vi "MaineReal.vi"() -> ()   [LabVIEW 2013]
panel:
  in  "AirmarVISAReference":refnum<visa-resource-name>="COM1"
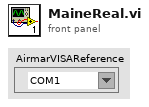
[diagram p1: front panel]
types:
  T1 = typedef "Notifiers.ctl" = cluster{"BoatSpeed":refnum<notifier>, "WindSpeed":refnum<notifier>, "MainPosition":refnum<notifier>, "JibPosition":refnum<notifier>, "MissionCheckOff":refnum<notifier>, "EStop":refnum<notifier>, "SpeedOverWater":refnum<notifier>, "BoatDirection":refnum<notifier>, "RudderPosition":refnum<notifier>, "Luffing":refnum<notifier>, "RudderForce":refnum<notifier>, "BatteryVoltage":refnum<notifier>, "StayForces":refnum<notifier>, "BoatLocation":refnum<notifier>}
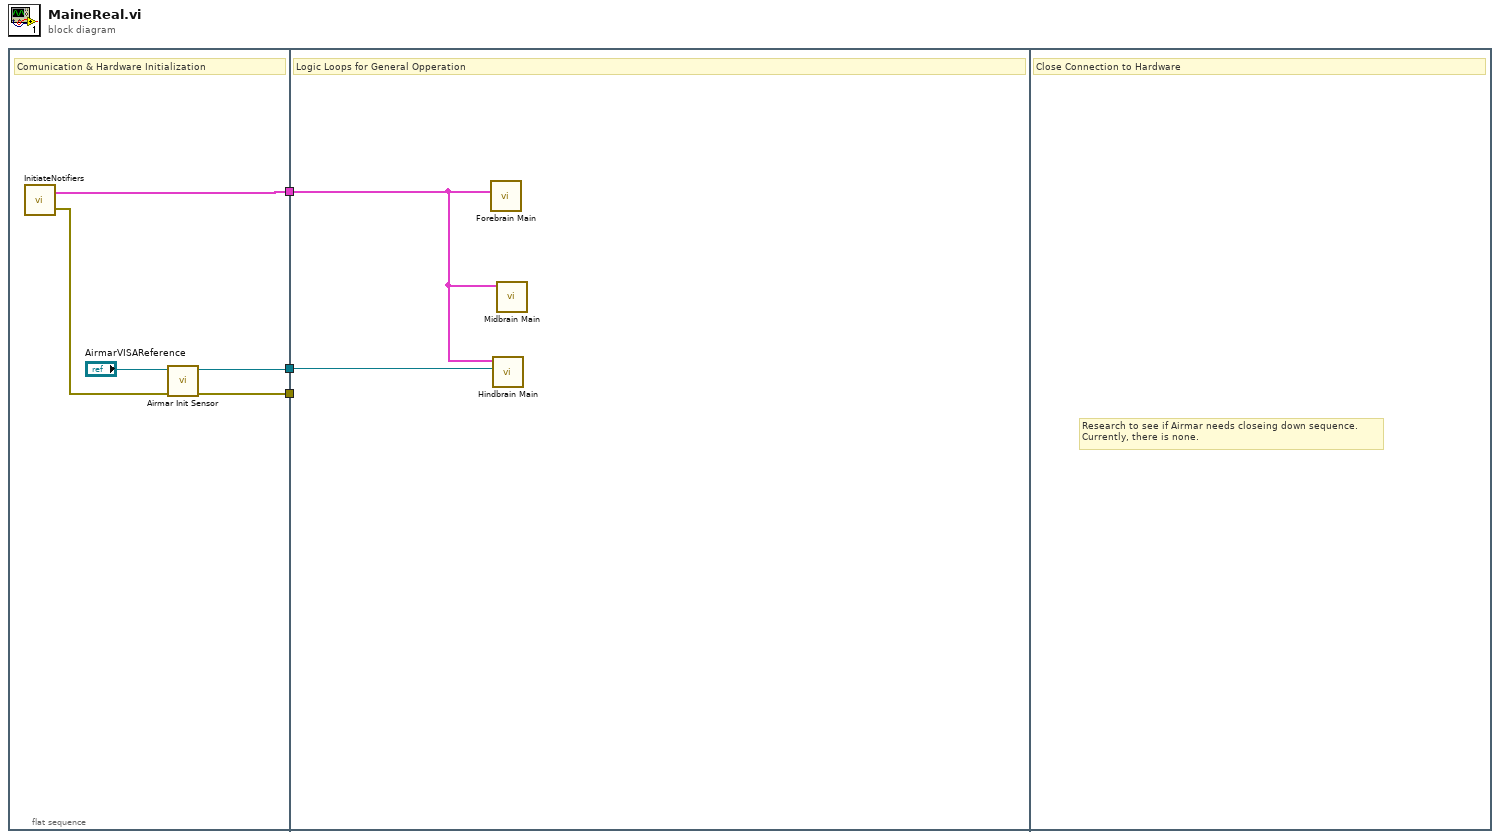
[diagram p0: block diagram]
diagram:
  n1 = flat-sequence {
    tunnel: [w8] -> w3
    tunnel: [w7] -> w2
    tunnel: [w4] -> w1
    tunnel: w3 -> [w10]
    tunnel: w2 -> [w9]
    tunnel: w1 -> [_]
    frame #0 {
      # "Comunication & Hardware Initialization"
      n2 = call "InitiateNotifiers.vi"() -> ("error out"=w5:errorcluster, "NotifierReferences"=w8:T1)  [unwired: 2 in]
      n3 = call "Airmar Init Sensor.vi"("error in (no error)"=w5, "VISA Refnum in"="AirmarVISAReference") -> ("error out"=w4:errorcluster, "VISA Refnum out"=w7:refnum<visa-resource-name>)  [unwired: 7 in, 1 out]
    }
    frame #1 {
      # "Logic Loops for General Opperation"
      n4 = call "Forebrain Main.vi"("NotifierReff"=w10) -> ()  [unwired: 3 in]
      n5 = call "Hindbrain Main.vi"("AirmarVISARefference"=w9, "NotifierReff"=w10) -> ()  [unwired: 10 in]
      n6 = call "Midbrain Main.vi"("NotifierReff"=w10) -> ()  [unwired: 11 in]
    }
    frame #2 {
      # "Research to see if Airmar needs closeing down sequence.\nCurrently, there is none."
      # "Close Connection to Hardware"
    }
  }
